vi "Stop.vi"(7 "Pump ID (0:A)":T1, 8 "error in (no error)":errorcluster, 11 "VISA resource in":refnum<visa-resource-name>) -> (0 "error out":errorcluster, 3 "VISA resource out":refnum<visa-resource-name>)   [LabVIEW 2020, in "Global FIA milliGAT.lvlib"]
doc: "Stops the motion of the pump."
uses:
  <instrlib>/RxnRover/Global FIA milliGAT 3.14/Global FIA milliGAT.lvlib
  <instrlib>/RxnRover/Global FIA milliGAT 3.14/Public/Utility/Pump Address.ctl
  <instrlib>/RxnRover/Global FIA milliGAT 3.14/Private/Pump Parameter.ctl
panel:
  in  "Fast Stop (F)":bool
  # "Note\nIf the \"Fast Stop\" option is selected, Flow Acceleration\nis set to the Maximum Deceleration value.  Flow Acceleration\nmust be rest afterwards."
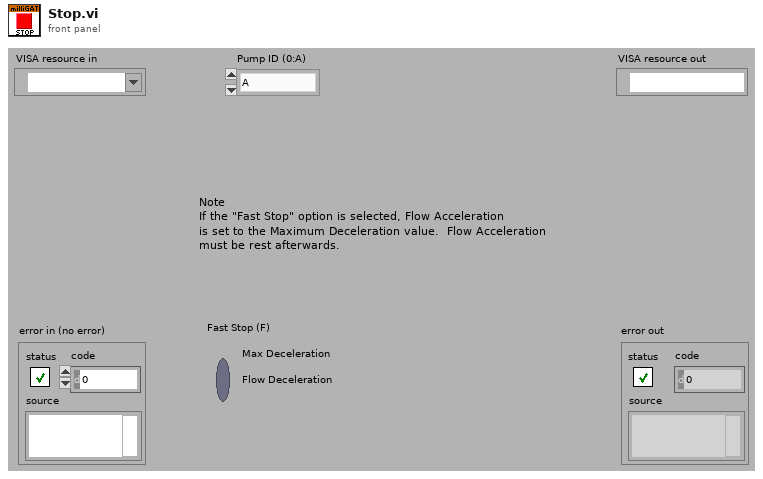
[diagram p1: front panel]
types:
  T1 = typedef "Global FIA milliGAT.lvlib/Pump Address.ctl" = enum16{"A", "B", "C", "D", "E", "F", "G", "H", "I", "J", "K", "L", "M", "N", "O", "P", "Q", "R", "S", "T", "U", "V", "W", "X", "Y", "Z", "a", "b", "c", "d", "e", "f", "g", "h", "i", "j", "k", "l", "m", "n", "o", "p", "q", "r", "s", "t", "u", "v", "w", "x", "y", "z", "0", "1", "2", "3", "4", "5", "6", "7", "8", "9"}
  T2 = typedef "Global FIA milliGAT.lvlib/Pump Parameter.ctl" = enum16{"Enabled", "EU", "EU Calibration Factor", "Fixed Asp or Disp", "Starting Position", "Starting Flow", "Peak Flow", "Flow Acceleration", "Flow Deceleration", "Session Volume", "Max Pressure", "Backlash (usteps)", "BL Calibration Factor", "BL Correction Enabled", "Min Flow", "Max Flow", "Min Acceleration", "Max Acceleration", "Service Volume", "Life Volume"}
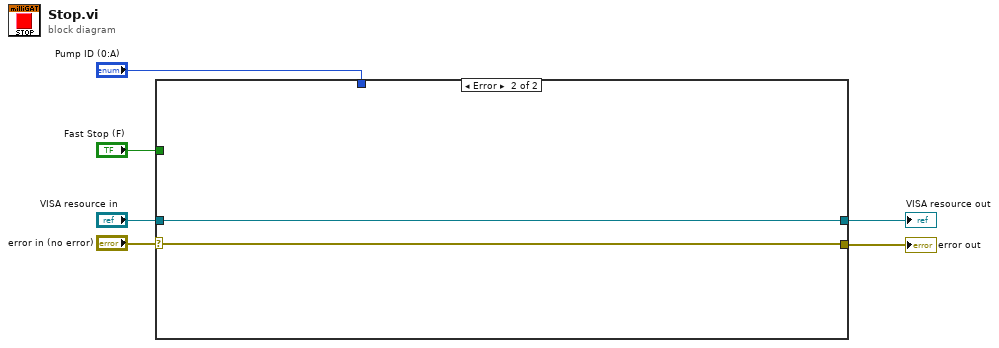
[diagram p0: block diagram]
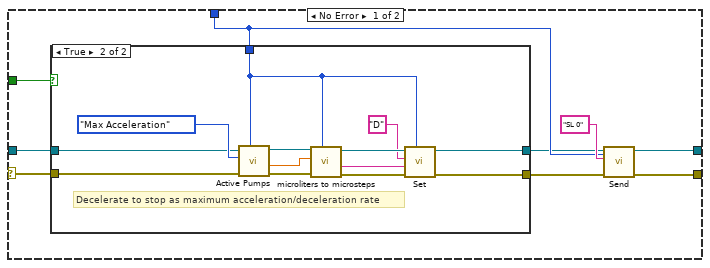
[diagram p2: hidden frame]
diagram:
  n1 = case shown="Error" "error in (no error)" {
    selector: "error in (no error)" -> [w7 w32]
    tunnel: "Pump ID (0:A)" -> [w14 _]
    tunnel: [w11 w31] -> w5
    tunnel: [w10 w32] -> w4
    tunnel: "VISA resource in" -> [w9 w31]
    tunnel: "Fast Stop (F)" -> [w8 _]
    frame No Error {
      n2 = case shown="True" w8 {
        tunnel: w14 -> [_ w26]
        tunnel: [w16 w22] -> w13
        tunnel: [w17 w21] -> w12
        tunnel: w9 -> [w17 w19]
        tunnel: w7 -> [w16 w18]
        frame False {
        }
        frame True {
          # "Decelerate to stop as maximum acceleration/deceleration rate"
          n3 = call <instrlib>:"Active Pumps.vi"("Pump ID (0:A)"=w26, "error in (no error)"=w18, "Parameter"=Pump_Parameter."Max Acceleration", "VISA resource in"=w19) -> ("error out"=w28:errorcluster, "Value out"=w20:dbl, "VISA resource out"=w29:refnum<visa-resource-name>)  [unwired: 4 in, 1 out]
          n4 = call <instrlib>:"microliters to microsteps.vi"("Pump ID (0:A)"=w26, "error in (no error)"=w28, "Microliters (0)"=w20, "VISA resource in"=w29) -> ("error out"=w23:errorcluster, "Microsteps (STR)"=w24:string, "VISA resource out"=w27:refnum<visa-resource-name>)  [unwired: 4 in, 1 out]
          n5 = call <instrlib>:"Set.vi"("Pump ID (0:A)"=w26, "error in (no error)"=w23, "Expression"=w24, "Parameter"="D", "VISA resource in"=w27) -> ("error out"=w22:errorcluster, "VISA resource out"=w21:refnum<visa-resource-name>)  [unwired: 5 in]
        }
      }
      n6 = call <instrlib>:"Send.vi"("Pump ID (0:A)"=w14, "error in (no error)"=w13, "Command"="SL 0" ("command"), "VISA resource in"=w12) -> ("error out"=w10:errorcluster, "VISA resource out"=w11:refnum<visa-resource-name>)  [unwired: 5 in, 1 out]
    }
    frame Error {
    }
  }
  "VISA resource out" <- w5
  "error out" <- w4
